vi "Data Read.vi"(6 "Append Index":i32, 8 "error in (no error)":errorcluster, 11 "path":path) -> (0 "error out":errorcluster, 1 "Notes":string, 2 "Data (Dictionary)":T1[](array[typedef]), 3 "path out":path)   [LabVIEW 2016, in "Data.lvclass"]
uses:
  Data.lvclass
  Typedefs/Dictionary--cluster.ctl
  Typedefs/Operation--enum.ctl
  Typedefs/File Type--enum.ctl
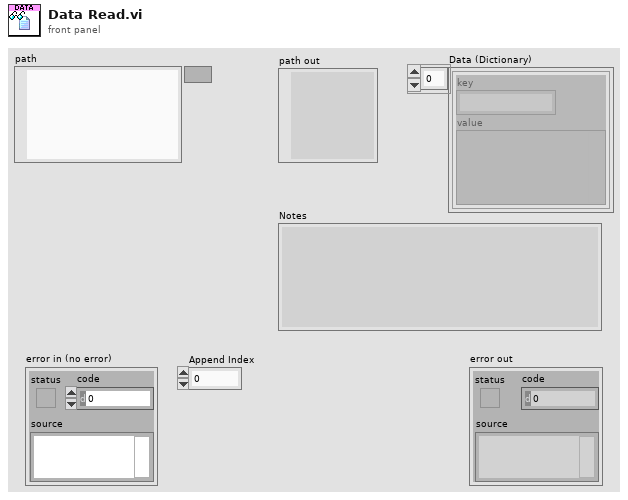
[diagram p1: front panel]
types:
  T1 = typedef "Data.lvclass/Dictionary--cluster.ctl" = cluster{"key":string, "value":variant}
  T2 = typedef "Data.lvclass/Operation--enum.ctl" = enum16{"Read", "Write", "Write + Append"}
  T3 = typedef "Data.lvclass/File Type--enum.ctl" = enum16{"DAT", "ITX", "HDF5", "TDMS", "VI", "PGSQL"}
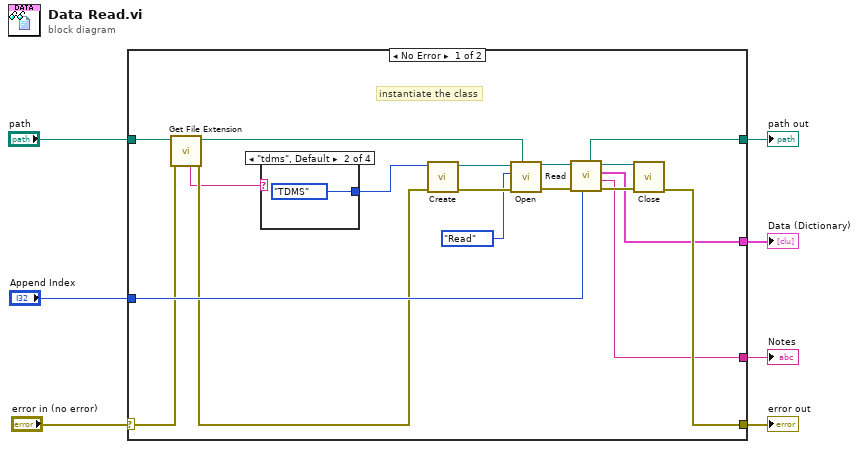
[diagram p0: block diagram]
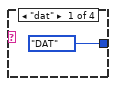
[diagram p2: hidden frame]
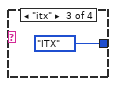
[diagram p3: hidden frame]
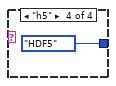
[diagram p4: hidden frame]
diagram:
  n1 = case shown="No Error" "error in (no error)" {
    selector: "error in (no error)" -> [w13 w31]
    tunnel: [w18 w31] -> w6
    tunnel: [w17 w30] -> w5
    tunnel: "path" -> [w11 w30]
    tunnel: [w16 _] -> w2
    tunnel: [w15 _] -> w3
    tunnel: "Append Index" -> [w14 _]
    frame No Error {
      # "instantiate the class"
      n2 = call <vilib>:"Get File Extension.vi"("error in (no error)"=w13, "file"=w11) -> ("error out"=w12:errorcluster, "dup file"=w10:path, "unmodified file extension"=w9:string)  [unwired: 5 in, 2 out]
      n3 = case shown="\"tdms\", Default" w9 {
        tunnel: [File_Type--enum."DAT" ("File Type") File_Type--enum."TDMS" ("File Type") File_Type--enum."ITX" ("File Type") File_Type--enum."HDF5" ("File Type")] -> w8
        frame "dat" {
        }
        frame "tdms", Default {
        }
        frame "itx" {
        }
        frame "h5" {
        }
      }
      n4 = call "Create.vi"("error in (no error)"=w12, "File Type"=w8) -> ("error out"=w24:errorcluster, "Data out"=w25:refnum<class "Data.lvclass">)  [unwired: 8 in]
      n5 = call-dynamic "Open.vi"("Path"=w10, "error in (no error)"=w24, "Operation"=Operation--enum."Read", "Data in"=w25) -> ("error out"=w22:errorcluster, "Data out"=w23:refnum<class "Data.lvclass">)  [unwired: 6 in]
      n6 = call-dynamic "Read.vi"("Append Index"=w14, "error in (no error)"=w22, "Data Save in"=w23) -> ("error out"=w20:errorcluster, "Notes"=w15:string, "Data (Dictionary)"=w16:T1[], "Data Save out"=w19:refnum<class "Data.lvclass">, "Path out"=w17:path)  [unwired: 4 in]
      n7 = call-dynamic "Close.vi"("error in (no error)"=w20, "Data in"=w19) -> ("error out"=w18:errorcluster)  [unwired: 8 in, 1 out]
    }
    frame Error {
    }
  }
  "error out" <- w6
  "path out" <- w5
  "Data (Dictionary)" <- w2
  "Notes" <- w3
